vi "Init.vi"(8 "error in (no error)":errorcluster, 9 "Config File Path":path=path "", 10 "Name":string, 11 "Report Generator In":refnum<class "Report Generator.lvclass">) -> (0 "error out":errorcluster, 3 "Report Generator Out":refnum<class "Report Generator.lvclass">)   [LabVIEW 2020, in "Report Generator.lvclass"]
uses:
  Report Generator.lvclass
  Report Classes/Plain Text Report/Plain Text Report.lvclass
  Application Framework/Process Classes/Process/Process.lvclass
  C:/Git/astemes-lunit/source/Framework/Report Classes/Test Report/Test Report.lvclass
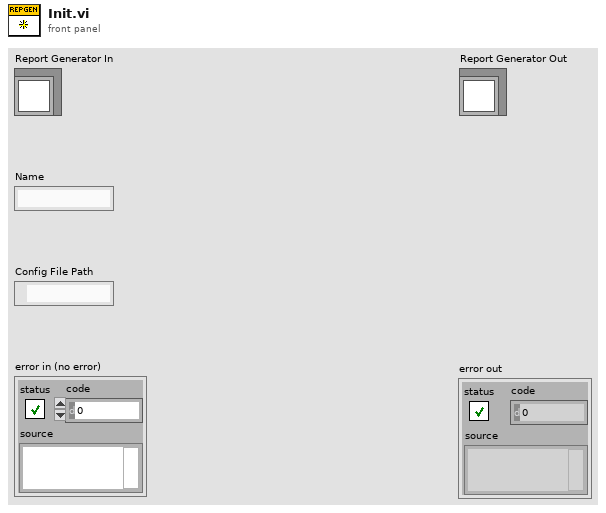
[diagram p1: front panel]
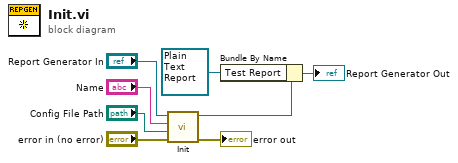
[diagram p0: block diagram]
diagram:
  n1 = call-parent "Init.vi"("error in (no error)"="error in (no error)", "Config File Path"="Config File Path", "Name"="Name", "Process In"="Report Generator In") -> ("error out"=→"error out":errorcluster, "Process Out"=w6:refnum<class "Report Generator.lvclass">)  [unwired: 6 in]
  n2 = Bundle By Name(cluster=w6, "Test Report"=refnum<class "Plain Text Report.lvclass"> refnum ("Plain Text Report.lvclass")) -> (→"Report Generator Out":refnum<class "Report Generator.lvclass">)
